vi "update waveform plot names.vi"(10 "selected plot names":string[](array[string]), 11 "WaveformChart in":refnum<vi>) -> ()   [LabVIEW 2016]
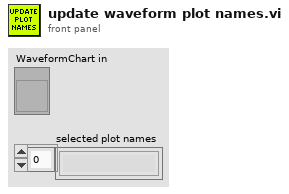
[diagram p1: front panel]
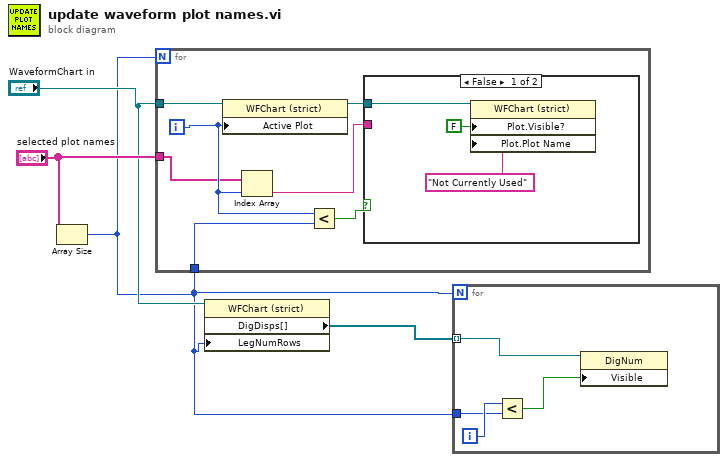
[diagram p0: block diagram]
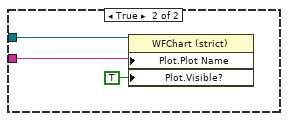
[diagram p2: hidden frame]
diagram:
  n1 = Array Size(array="selected plot names") -> (size(s)=w1:i32)
  n2 = for {
    N: w1 -> [_]
    tunnel: "WaveformChart in" -> [w11]
    tunnel: "selected plot names" -> [w6]
    tunnel: w1 -> [w9]
    i -> [w7]
    n3 = property class="WFChart (strict)"(reference=w11, "Active Plot"=w7) -> (reference out=w10:refnum<vi>)  [unwired: 1 in, 1 out]
    n4 = Index Array(array=w6, index=w7) -> (element=w5:string)
    n5 = Less?(x=w7, y=w9) -> (x < y?=w8:bool)
    n6 = case shown="False" w8 {
      tunnel: w10 -> [w14 w17]
      tunnel: w5 -> [_ w16]
      frame False {
        n7 = property class="WFChart (strict)"(reference=w14, "Plot.Visible?"=FALSE ("Plot.Visible"), "Plot.Plot Name"="Not Currently Used") -> ()  [unwired: 1 in, 2 out]
      }
      frame True {
        n8 = property class="WFChart (strict)"(reference=w17, "Plot.Plot Name"=w16, "Plot.Visible?"=TRUE ("Plot.Visible")) -> ()  [unwired: 1 in, 2 out]
      }
    }
  }
  n9 = property class="WFChart (strict)"(reference="WaveformChart in", "LegNumRows"=w1) -> ("DigDisps[]"=w3:refnum<vi>[])  [unwired: 1 in, 2 out]
  n10 = for {
    N: w1 -> [_]
    tunnel: w3 -> [w21] mode=indexing
    tunnel: w1 -> [w19]
    i -> [w20]
    n11 = Less?(x=w20, y=w19) -> (x < y?=w18:bool)
    n12 = property class="DigNum"(reference=w21, "Visible"=w18) -> ()  [unwired: 1 in, 2 out]
  }
